vi "Base Card Passthrough(Properties).vi"(4 "Iterations":u32=50 min=1 max=64, 6 "Channels (1-64)":u16=64 min=1 max=64, 11 "device":refnum<k21>="SET-2010-Mod2") -> (0 "error out":errorcluster, 1 "Disconnect Timing":T1, 2 "Connect Timing":T1)   [LabVIEW 2020, in "slsc-switch-benchmarks.lvlib"]
uses:
  slsc-switch-benchmarks.lvlib
  Timing Statistics.ctl
  <vilib>/SLSC/Initialize Session with Devices.vi
  <vilib>/SLSC/Set Phys Chan Property (Bool).vi
  <vilib>/SLSC/Commit Properties for Devices.vi
  <vilib>/SLSC/Close Session.vi
  <vilib>/SLSC/SLSC.lvlib
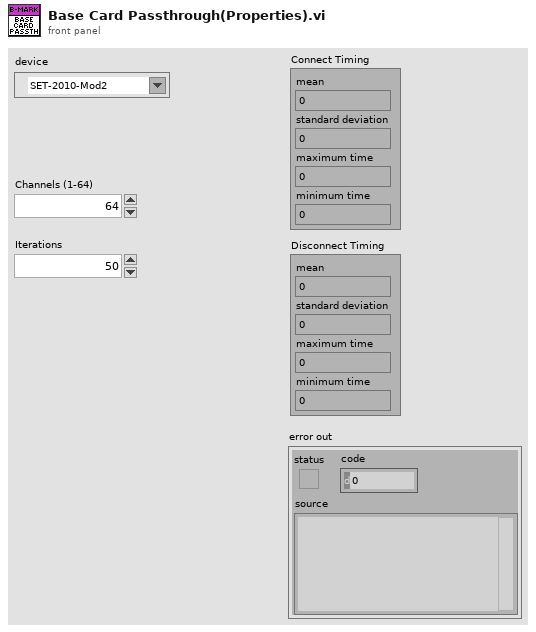
[diagram p1: front panel]
types:
  T1 = typedef "slsc-switch-benchmarks.lvlib/Timing Statistics.ctl" = cluster{"mean":dbl, "standard deviation":dbl, "maximum time":dbl, "minimum time":dbl}
  T2 = cluster{"Connect Time":dbl, "Disconnect Time":dbl}
  T3 = cluster{"Connect Time":dbl, "Disconnect Time":dbl}[]
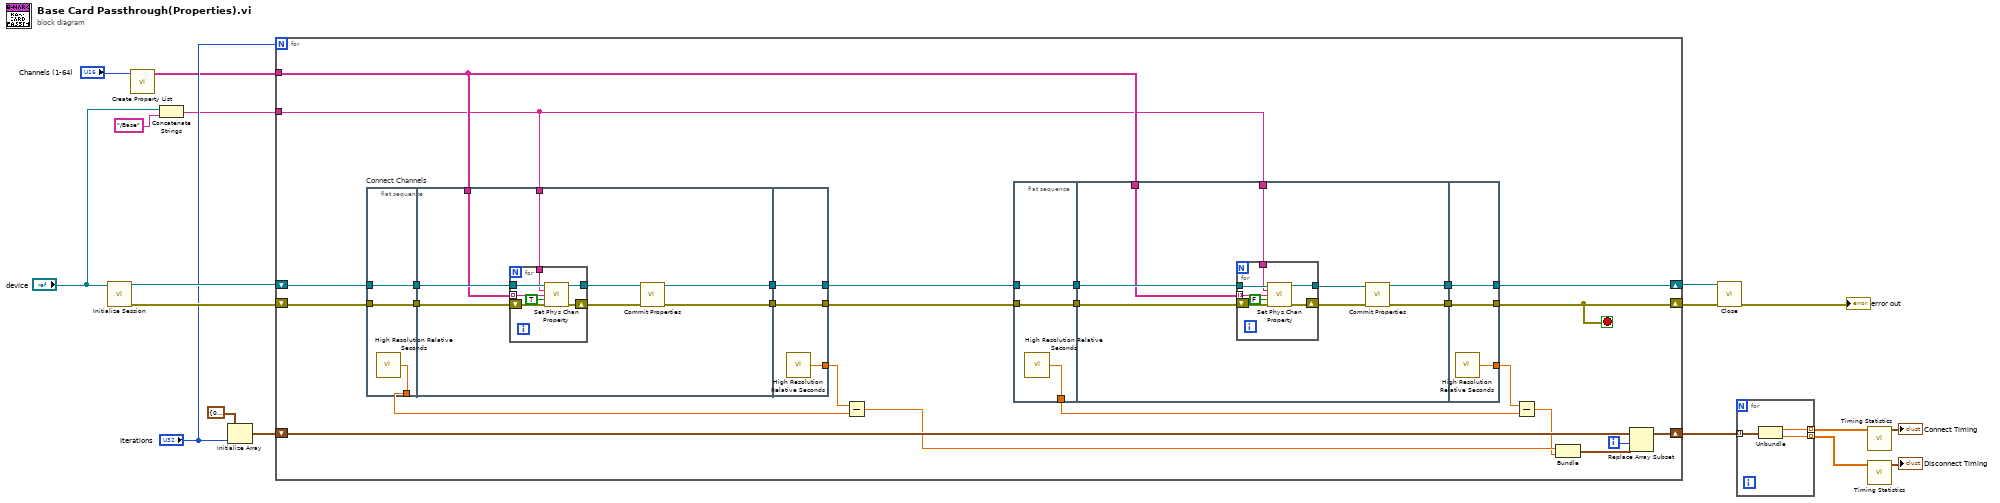
[diagram p0: block diagram]
diagram:
  n1 = call-poly <vilib>:"Initialize Session.vi"("devices"="device") -> ("session out"=w12:refnum<k21>, "error out"=w11:errorcluster)  [unwired: 13 in]
  n2 = call "Create Property List.vi"("Channels (1-64)"="Channels (1-64)") -> ("Property List"=w4:string[])  [unwired: 10 in]
  n3 = Concatenate Strings("device", "/Base") -> (w1:string)
  n4 = Initialize Array(T2 {"Connect Time"=0.0, "Disconnect Time"=0.0}, "Iterations") -> (w18:T3)
  n5 = for {
    N: "Iterations" -> [_]
    shift-right: [w40] -> w9
    shift-left: w12 -> [w44]
    shift-right: [w27] -> w10
    shift-left: w11 -> [w43]
    shift-right: [w24] -> w17
    shift-left: w18 -> [w25]
    tunnel: w4 -> [w20]
    tunnel: w1 -> [w19]
    i -> [w26]
    stop <- w27 stop-if-true
    n6 = flat-sequence "Connect Channels" {
      tunnel: w43 -> [w67]
      tunnel: w44 -> [w68]
      tunnel: [w68] -> w37
      tunnel: [w67] -> w36
      tunnel: [w66] -> w34
      tunnel: [w70] -> w39
      tunnel: [w69] -> w38
      tunnel: w37 -> [w76]
      tunnel: w36 -> [w75]
      tunnel: w20 -> [w74]
      tunnel: w19 -> [w73]
      tunnel: [w85] -> w41
      tunnel: [w86] -> w42
      tunnel: w39 -> [w86]
      tunnel: w38 -> [w85]
      tunnel: [w84] -> w35
      frame #0 {
        n7 = call <vilib>:"High Resolution Relative Seconds.vi"() -> ("relative seconds"=w66:dbl)
      }
      frame #1 {
        n8 = for {
          shift-right: [w81] -> w71
          shift-left: w75 -> [w80]
          tunnel: w76 -> [w83]
          tunnel: [w82] -> w72
          tunnel: w74 -> [w79] mode=indexing
          tunnel: w73 -> [w77]
          n9 = call-poly <vilib>:"Set Phys Chan Property.vi"("session in"=w83, "physical channels"=w77, "property"=w79, "property value"=TRUE, "error in (no error)"=w80) -> ("session out"=w82:refnum<k21>, "error out"=w81:errorcluster)  [unwired: 9 in]
        }
        n10 = call-poly <vilib>:"Commit Properties.vi"("session in"=w72, "error in (no error)"=w71) -> ("session out"=w70:refnum<k21>, "error out"=w69:errorcluster)  [unwired: 12 in]
      }
      frame #2 {
        n11 = call <vilib>:"High Resolution Relative Seconds.vi"() -> ("relative seconds"=w84:dbl)
      }
    }
    n12 = Subtract(x=w35, y=w34) -> (x-y=w23:dbl)
    n13 = flat-sequence {
      tunnel: w41 -> [w46]
      tunnel: w42 -> [w47]
      tunnel: [w47] -> w33
      tunnel: [w46] -> w32
      tunnel: [w45] -> w28
      tunnel: w33 -> [w55]
      tunnel: w32 -> [w54]
      tunnel: [w49] -> w31
      tunnel: [w48] -> w30
      tunnel: w20 -> [w53]
      tunnel: w19 -> [w52]
      tunnel: [w64] -> w40
      tunnel: [w65] -> w27
      tunnel: w31 -> [w65]
      tunnel: w30 -> [w64]
      tunnel: [w63] -> w29
      frame #0 {
        n14 = call <vilib>:"High Resolution Relative Seconds.vi"() -> ("relative seconds"=w45:dbl)
      }
      frame #1 {
        n15 = for {
          shift-right: [w60] -> w50
          shift-left: w54 -> [w61]
          tunnel: w55 -> [w62]
          tunnel: [w59] -> w51
          tunnel: w53 -> [w58] mode=indexing
          tunnel: w52 -> [w56]
          n16 = call-poly <vilib>:"Set Phys Chan Property.vi"("session in"=w62, "physical channels"=w56, "property"=w58, "property value"=FALSE, "error in (no error)"=w61) -> ("session out"=w59:refnum<k21>, "error out"=w60:errorcluster)  [unwired: 9 in]
        }
        n17 = call-poly <vilib>:"Commit Properties.vi"("session in"=w51, "error in (no error)"=w50) -> ("session out"=w48:refnum<k21>, "error out"=w49:errorcluster)  [unwired: 12 in]
      }
      frame #2 {
        n18 = call <vilib>:"High Resolution Relative Seconds.vi"() -> ("relative seconds"=w63:dbl)
      }
    }
    n19 = Subtract(x=w29, y=w28) -> (x-y=w22:dbl)
    n20 = Bundle(w23, w22) -> (w21:cluster{dbl, dbl})  [unwired: 1 in]
    n21 = Replace Array Subset(array=w25, new element=w21, index=w26) -> (w24:T3)
  }
  n22 = call-poly <vilib>:"Close.vi"("session in"=w9, "error in (no error)"=w10) -> ("error out"=→"error out":errorcluster)  [unwired: 13 in]
  n23 = for {
    tunnel: w17 -> [w89] mode=indexing
    tunnel: [w88] -> w16 mode=indexing
    tunnel: [w87] -> w15 mode=indexing
    n24 = Unbundle(w89) -> ("Connect Time"=w88:dbl, "Disconnect Time"=w87:dbl)
  }
  n25 = call "Timing Statistics.vi"("Execution Speeds"=w16) -> ("Timing Statistics"=→"Connect Timing":T1)  [unwired: 10 in]
  n26 = call "Timing Statistics.vi"("Execution Speeds"=w15) -> ("Timing Statistics"=→"Disconnect Timing":T1)  [unwired: 10 in]
